vi "ConvertBufferToString.vi"(10 "Buffer":u8=1 min=1 max=2 step=1, 11 "SMU":T1) -> (3 "Buffer":string)   [LabVIEW 2012, in "Keithley-2602.lvlib"]
uses:
  Keithley-2602.lvlib
  Public/Controls/SMU.ctl
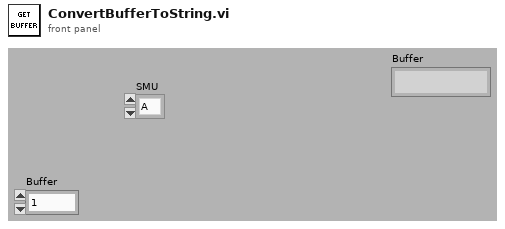
[diagram p1: front panel]
types:
  T1 = typedef "Keithley-2602.lvlib/SMU.ctl" = enum16{"A", "B"}
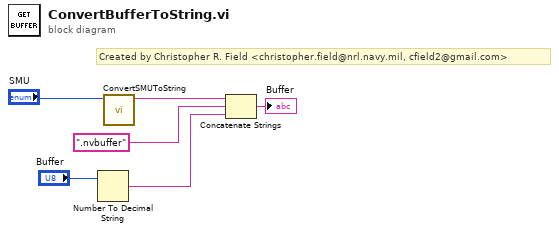
[diagram p0: block diagram]
diagram:
  # "Created by Christopher R. Field <christopher.field@nrl.navy.mil, cfield2@gmail.com>"
  n1 = Number To Decimal String(number="Buffer") -> (decimal integer string=w3:string)  [unwired: 1 in]
  n2 = call "ConvertSMUToString.vi"("SMU"="SMU") -> ("Channel"=w6:string)  [unwired: 10 in]
  n3 = Concatenate Strings(w6, ".nvbuffer" ("string"), w3) -> (→"Buffer":string)
